vi "Configure DC Voltage.vi"(0 "VISA resource name":refnum<visa-resource-name>, 5 "Output DC Voltage (115 V)":dbl=115.0 min=0.0 max=400.0 format="%.1f", 11 "error in (no error)":errorcluster) -> (4 "VISA resource name out":refnum<visa-resource-name>, 15 "error out":errorcluster)   [LabVIEW 2016, in "APT 300XAC Series.lvlib"]
doc: "Sets the <B>DC Voltage</B> in the active step of the power source instrument.\n\nThe voltage parameter setting configures the voltage output.\nIn the DC+/DC- mode the operator can select either a positive or negative DC output. This selection will only be available if the DC option has been installed on the AC power source insrument.\nVoltage is the amount of force that is needed to move current from point to point."
uses:
  APT 300XAC Series.lvlib
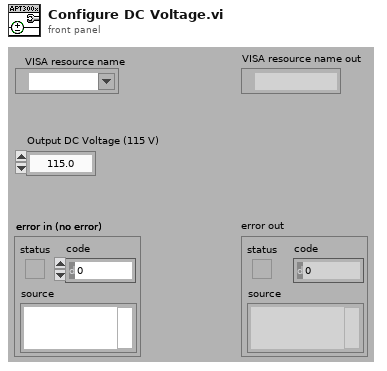
[diagram p1: front panel]
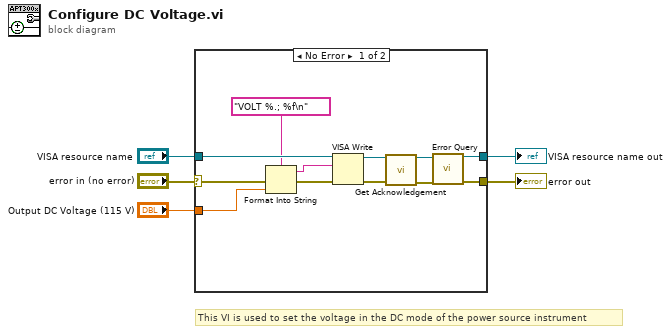
[diagram p0: block diagram]
diagram:
  # "This VI is used to set the voltage in the DC mode of the power source instrument"
  n1 = case shown="No Error" "error in (no error)" {
    selector: "error in (no error)" -> [w11 w19]
    tunnel: "VISA resource name" -> [w17 w18]
    tunnel: [w13 w18] -> w4
    tunnel: [w12 w19] -> w3
    tunnel: "Output DC Voltage (115 V)" -> [w15 _]
    frame No Error {
      n2 = Format Into String(format string="VOLT %.; %f\n" ("Command"), error in=w11, w15) -> (resulting string=w14:string, error out=w10:errorcluster)  [unwired: 1 in]
      n3 = VISA Write(VISA resource name=w17, write buffer=w14, error in (no error)=w10) -> (VISA resource name out=w9:refnum<visa-resource-name>, error out=w7:errorcluster)  [unwired: 1 out]
      n4 = call "Get Acknowledgement.vi"("VISA resource name"=w9, "error in (no error)"=w7) -> ("VISA resource name out"=w8:refnum<visa-resource-name>, "error out"=w6:errorcluster)  [unwired: 12 in]
      n5 = call "Error Query.vi"("VISA resource name"=w8, "error in (no error)"=w6) -> ("VISA resource name out"=w13:refnum<visa-resource-name>, "error out"=w12:errorcluster)  [unwired: 10 in, 2 out]
    }
    frame Error {
    }
  }
  "error out" <- w3
  "VISA resource name out" <- w4
